vi "Disconnect.vi"(0 "Location of FieldMax2Lib.dll in":path=path "C:/Windows/System32/FieldMax2Lib.dll", 1 "Meter ID in":i32, 3 "error in (no error)":errorcluster) -> (7 "Location of FieldMax2Lib.dll out":path, 8 "Meter ID out":i32, 10 "error out":errorcluster)   [LabVIEW 2012]
panel:
  # "This VI should be run at the end of the routine to close communications with the meter."
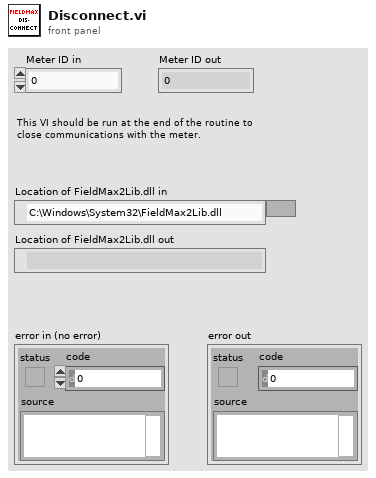
[diagram p1: front panel]
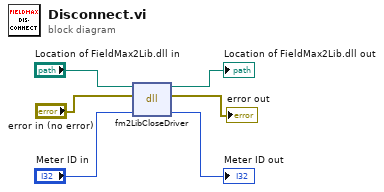
[diagram p0: block diagram]
diagram:
  n1 = dll-call lib="C:/Windows/System32/FieldMax2Lib.dll" fn="fm2LibCloseDriver" label="Close Driver"(path in="Location of FieldMax2Lib.dll in", error in="error in (no error)", "h"="Meter ID in") -> (path out=→"Location of FieldMax2Lib.dll out":path, error out=→"error out":errorcluster, "h"=→"Meter ID out":i32)  [unwired: 2 in]
